vi "from string.vi"(8 "error in":errorcluster, 9 "data":string, 10 "version":string, 11 "configuration in":refnum<class "action configuration.lvclass">) -> (0 "error out":errorcluster, 3 "configuration out":refnum<class "action configuration.lvclass">)   [LabVIEW 2014, in "action configuration.lvclass"]
doc: "Provides an interface for loading a module configuration from a file or other serialized data source. It is recommended that all children of this class store data in two sets--data required for its own initialization, and any data required for parent initialization--and that each implementation uses the <b>Call Parent Method</b> primitive to de-serialize parent information."
uses:
  action configuration.lvclass
  <vilib>/NI/Tag Bus Module Framework/root configuration/TBM configuration.lvclass
  <vilib>/NI/Configuration Framework/serializable configuration/NISE_CEF_serializable configuration.lvclass
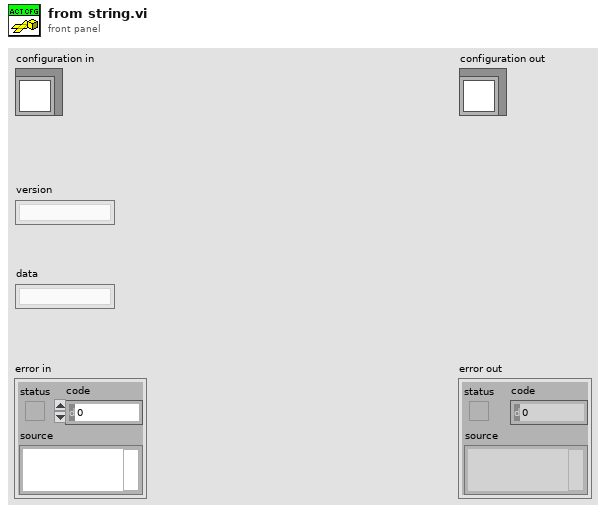
[diagram p1: front panel]
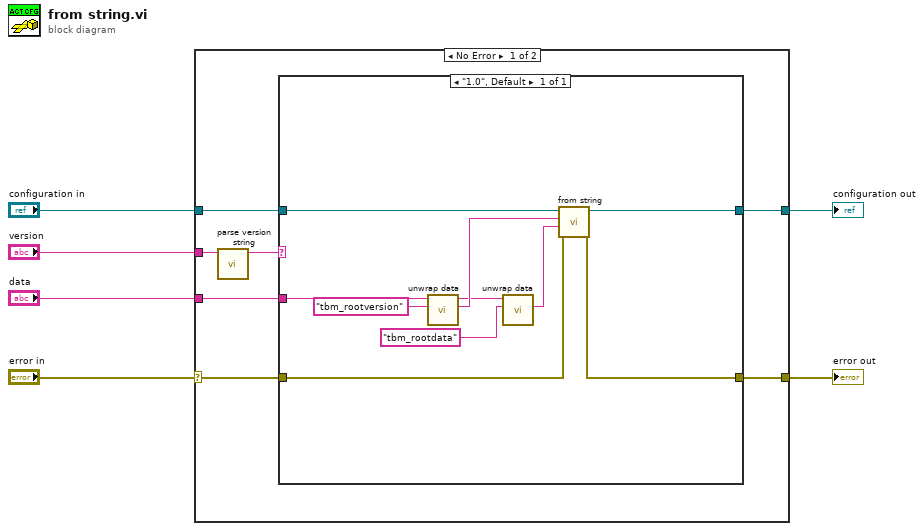
[diagram p0: block diagram]
diagram:
  n1 = case shown="No Error" "error in" {
    selector: "error in" -> [w11 w24]
    tunnel: "configuration in" -> [w13 w25]
    tunnel: "version" -> [w8 _]
    tunnel: "data" -> [w12 _]
    tunnel: [w10 w24] -> w2
    tunnel: [w9 w25] -> w1
    frame No Error {
      n2 = call <vilib>:"parse version string.vi"("full version"=w8) -> ("major.minor version"=w7:string)  [unwired: 7 in, 3 out]
      n3 = case shown="\"1.0\", Default" w7 {
        tunnel: w13 -> [w23]
        tunnel: w12 -> [w19]
        tunnel: w11 -> [w22]
        tunnel: [w21] -> w10
        tunnel: [w20] -> w9
        frame "1.0", Default {
          n4 = call <vilib>:"unwrap data.vi"("identifier"="tbm_rootversion" ("additional identifier"), "data to unwrap"=w19) -> ("unwrapped data"=w17:string, "remaining string"=w16:string)  [unwired: 8 in]
          n5 = call <vilib>:"unwrap data.vi"("identifier"="tbm_rootdata" ("additional identifier"), "data to unwrap"=w16) -> ("unwrapped data"=w14:string)  [unwired: 8 in, 1 out]
          n6 = call-parent "from string.vi"("error in"=w22, "data"=w14, "version"=w17, "configuration in"=w23) -> ("error out"=w21:errorcluster, "configuration out"=w20:refnum<class "action configuration.lvclass">)  [unwired: 6 in]
        }
      }
    }
    frame Error {
    }
  }
  "error out" <- w2
  "configuration out" <- w1
